vi "StringProbe.vi"(11 "PriorityQueue out":refnum<class "PriorityQueue.lvclass">) -> (2 "Value String":string, 3 "Boolean":bool)   [LabVIEW 2019, in "PriorityQueue.lvclass"]
uses:
  PriorityQueue.lvclass
  PriorityQueue.lvclass/PriorityQueue.ctl
panel:
  out "Array":string[](array[string])
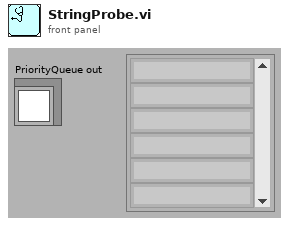
[diagram p1: front panel]
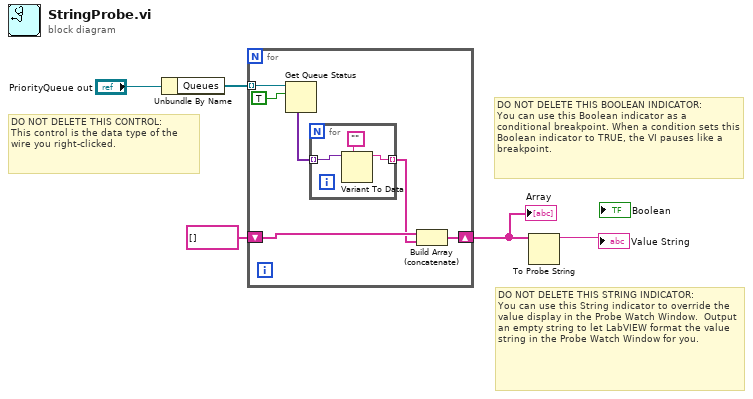
[diagram p0: block diagram]
diagram:
  # "DO NOT DELETE THIS STRING INDICATOR: \nYou can use this String indicator to override the value display in the Probe Watch Window.  Output an empty string to let LabVIEW format the value string in the Probe Watch Window for you."
  # "DO NOT DELETE THIS BOOLEAN INDICATOR: \nYou can use this Boolean indicator as a conditional breakpoint. When a condition sets this Boolean indicator to TRUE, the VI pauses like a breakpoint."
  # "DO NOT DELETE THIS CONTROL: \nThis control is the data type of the wire you right-clicked."
  n1 = Unbundle By Name("PriorityQueue out") -> ("Queues"=w3:refnum<queue>[])
  n2 = for {
    tunnel: w3 -> [w11] mode=indexing
    shift-right: [w9] -> w1
    shift-left: string[] [] -> [w8]
    n3 = Get Queue Status(queue=w11, return elements? (F)=TRUE) -> (elements=w7:variant[])  [unwired: 1 in, 7 out]
    n4 = for {
      tunnel: w7 -> [w14] mode=indexing
      tunnel: [w12] -> w6 mode=indexing
      n5 = Variant To Data(type="", Variant=w14) -> (data=w12:string)  [unwired: 1 in, 1 out]
    }
    n6 = Build Array (concatenate)(w8, w6) -> (w9:string[])
  }
  "Array" <- w1
  n7 = To Probe String(7:w1) -> (3:→"Value String":string)  [unwired: 2 in, 1 out]
